vi "Get Label.vi"(8 "error in (no error)":errorcluster, 11 "Hardware.lvlib:CCD.lvlib:CCD Configuration.lvclass":refnum<class "CCD Configuration.lvclass">) -> (0 "error out":errorcluster, 2 "Label":string, 3 "Hardware.lvlib:CCD.lvlib:CCD Configuration.lvclass 2":refnum<class "CCD Configuration.lvclass">)   [LabVIEW 2016, in "CCD.lvlib" / "CCD Configuration.lvclass"]
uses:
  <userlib>/Common Components/Hardware/CCD/CCD Configuration.lvclass
  <userlib>/Common Components/Hardware/CCD/CCD Configuration.lvclass/CCD Configuration.ctl
  <userlib>/Common Components/Hardware/Abstract Hardware/Hardware.lvclass/Hardware.ctl
  <userlib>/Common Components/Hardware/Abstract Hardware/Read Label.vi
  <userlib>/Common Components/Hardware/CCD/CCD/CCD.lvclass
  C:/Program Files (x86)/National Instruments/LabVIEW 2016/user.lib/Common Components/Hardware/Abstract Hardware/Hardware.lvclass
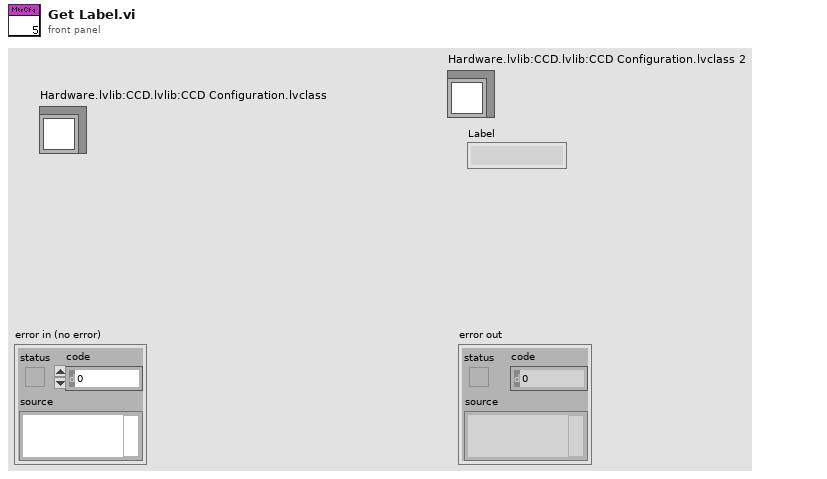
[diagram p1: front panel]
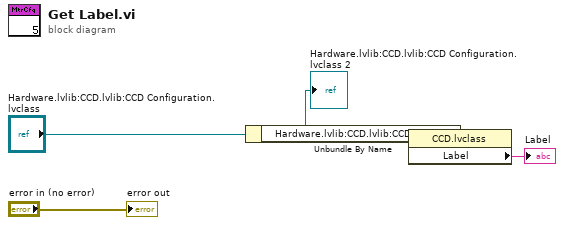
[diagram p0: block diagram]
diagram:
  n1 = Unbundle By Name("Hardware.lvlib:CCD.lvlib:CCD Configuration.lvclass") -> ("Hardware.lvlib:CCD.lvlib:CCD.lvclass"=w3:refnum<class "CCD.lvclass">)
  n2 = property class="CCD.lvclass"(reference=w3) -> ("Label"=→"Label":string)  [unwired: 1 in, 2 out]
  "error out" <- "error in (no error)"
  "Hardware.lvlib:CCD.lvlib:CCD Configuration.lvclass 2" <- "Hardware.lvlib:CCD.lvlib:CCD Configuration.lvclass"
